vi "Read Measurement.vi"   [LabVIEW 2017, in "Keysight B2980 Series.lvlib"]
doc: "Read the measurement result."
uses:
  Keysight B2980 Series.lvlib
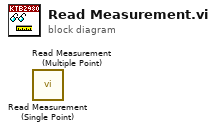
[diagram p0: block diagram]
diagram:
  n1 = call "Read Measurement (Single Point).vi"() -> ()  [unwired: 9 in, 3 out]
  n2 = call "Read Measurement (Multiple Point).vi"() -> ()  [unwired: 9 in, 3 out]
